vi "Daxsonics Read Write.vi"(7 "Daxsonics Name":T1=enum."New2021", 8 "error IN":errorcluster, 10 "write buffer":string, 11 "VISA resource name":refnum<visa-resource-name>="ASRL4::INSTR") -> (0 "error out":errorcluster, 1 "Success?":bool, 2 "read buffer":string)   [LabVIEW 2022 SP3]
uses:
  Daxsonics_Pulsers.ctl
  <vilib>/Instr/_visa.llb/VISA Configure Serial Port (Instr).vi
panel:
  # ":BEAM:PRI?"
  # ":BEAM:NUMTX?"
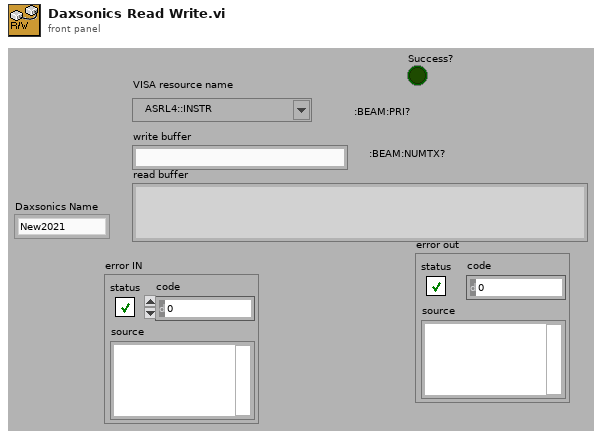
[diagram p1: front panel]
types:
  T1 = typedef "Daxsonics_Pulsers.ctl" = enum16{"BP1", "BP2_A", "BP2_B", "10ERS8", "New2021"}
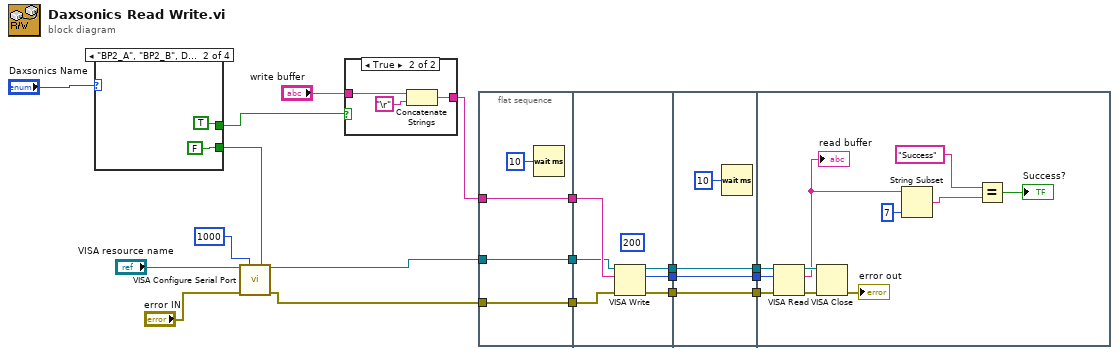
[diagram p0: block diagram]
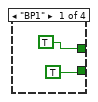
[diagram p2: hidden frame]
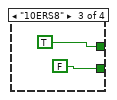
[diagram p3: hidden frame]
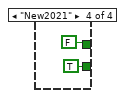
[diagram p4: hidden frame]
diagram:
  n1 = case shown="\"BP2_A\", \"BP2_B\", Default" "Daxsonics Name" {
    tunnel: [TRUE ("Enable Termination\nChar (T)") FALSE ("Enable Termination\nChar (T)") FALSE ("Enable Termination\nChar (T)") TRUE ("CR on Write?")] -> w13
    tunnel: [TRUE ("Enable Termination\nChar (T)") TRUE ("Enable Termination\nChar (T)") TRUE ("Enable Termination\nChar (T)") FALSE ("CR on Write?")] -> w14
    frame "BP1" {
    }
    frame "BP2_A", "BP2_B", Default {
    }
    frame "10ERS8" {
    }
    frame "New2021" {
    }
  }
  n2 = call-poly "VISA Configure Serial Port"("VISA resource name"="VISA resource name", "timeout (10sec)"=u32 1000, "Enable Termination\nChar (T)"=w13, "error in (no error)"="error IN") -> ("VISA resource name out"=w4:refnum<visa-resource-name>, "error out"=w6:errorcluster)  [unwired: 10 in]
  n3 = case shown="True" w14 {
    tunnel: "write buffer" -> [w28 w30]
    tunnel: [w28 w29] -> w5
    frame False {
    }
    frame True {
      n4 = Concatenate Strings(w30, "\r") -> (w29:string)
    }
  }
  n5 = flat-sequence {
    tunnel: w4 -> [w33]
    tunnel: w5 -> [w34]
    tunnel: w6 -> [w35]
    tunnel: [w35] -> w3
    tunnel: [w34] -> w2
    tunnel: [w33] -> w1
    tunnel: [w36] -> w12
    tunnel: [w38] -> w10
    tunnel: [w37] -> w8
    tunnel: w3 -> [w41]
    tunnel: w2 -> [w40]
    tunnel: w1 -> [w39]
    tunnel: w12 -> [w45]
    tunnel: [w45] -> w11
    tunnel: w10 -> [w44]
    tunnel: [w44] -> w9
    tunnel: w8 -> [w43]
    tunnel: [w43] -> w7
    tunnel: w11 -> [w53]
    tunnel: w9 -> [w52]
    tunnel: w7 -> [w51]
    frame #0 {
      n6 = Wait (ms)(milliseconds to wait=u32 10) -> ()  [unwired: 1 out]
    }
    frame #1 {
      (unwired) u32 200 ("byte count")
      n7 = VISA Write(VISA resource name=w39, write buffer=w40, error in (no error)=w41) -> (VISA resource name out=w36:refnum<visa-resource-name>, return count=w37:u32, error out=w38:errorcluster)
    }
    frame #2 {
      n8 = Wait (ms)(milliseconds to wait=u32 10) -> ()  [unwired: 1 out]
    }
    frame #3 {
      n9 = VISA Read(VISA resource name=w53, byte count=w51, error in (no error)=w52) -> (VISA resource name out=w56:refnum<visa-resource-name>, read buffer=w48:string, error out=w55:errorcluster)  [unwired: 1 out]
      "read buffer" <- w48
      n10 = VISA Close(VISA resource name=w56, error in (no error)=w55) -> (error out=→"error out":errorcluster)
      n11 = String Subset(string=w48, length (rest)=7 ("length (rest)")) -> (substring=w49:string)  [unwired: 1 in]
      n12 = Equal?(x="Success", y=w49) -> (x = y?=→"Success?":bool)
    }
  }
